vi "execute.vi"(8 "error in (no error)":errorcluster, 10 "Context in":refnum<class "Context.lvclass">, 11 "ExitMaintenanceCommand in":refnum<class "ExitMaintenanceCommand.lvclass">) -> (0 "error out":errorcluster, 2 "Context out":refnum<class "Context.lvclass">, 3 "ExitMaintenanceCommand out":refnum<class "ExitMaintenanceCommand.lvclass">)   [LabVIEW 2016, in "ExitMaintenanceCommand.lvclass"]
uses:
  ExitMaintenanceCommand.lvclass
  Context/Context.lvclass
  ExitMaintenanceCommand.lvclass/ExitMaintenanceCommand.ctl
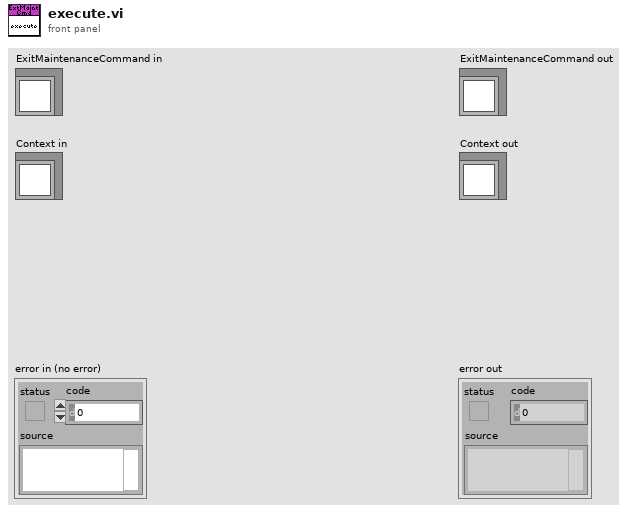
[diagram p1: front panel]
types:
  T1 = typedef "M1M3SupportTopics.lvlib/CommandExitMaintenance.ctl" = cluster{"CommandId":T2, "ExitMaintenance":bool}
  T2 = typedef "M1M3SupportTopics.lvlib/CommandId.ctl" = i32
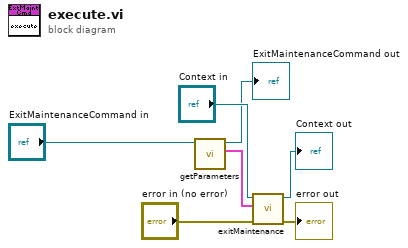
[diagram p0: block diagram]
diagram:
  n1 = call "getParameters.vi"("ExitMaintenanceCommand in"="ExitMaintenanceCommand in") -> ("Parameters"=w5:T1, "ExitMaintenanceCommand out"=→"ExitMaintenanceCommand out":refnum<class "ExitMaintenanceCommand.lvclass">)  [unwired: 9 in]
  n2 = call "exitMaintenance.vi"("error in (no error)"="error in (no error)", "Parameters"=w5, "Context in"="Context in") -> ("error out"=→"error out":errorcluster, "Context out"=→"Context out":refnum<class "Context.lvclass">)  [unwired: 7 in]
